vi "Window Coefficients.vi"(1 "window type":T1(ring)=enum."Hanning", 2 "window length":i32=1024) -> (0 "coefficients":dbl[](array[numeric]) format="%.2f")   [LabVIEW 2017]
uses:
  <vilib>/Analysis/4window.llb/Blackman Window (DBL).vi
  <vilib>/Analysis/4window.llb/Hamming Window (DBL).vi
  <vilib>/Analysis/4window.llb/Hanning Window (DBL).vi
  <vilib>/Analysis/baseanly.llb/Unit Vector (DBL).vi
  <vilib>/Analysis/4window.llb/AllCosWindow (DBL).vi
  <vilib>/Analysis/NI_AALBase.lvlib
  <vilib>/Analysis/NI_AALPro.lvlib
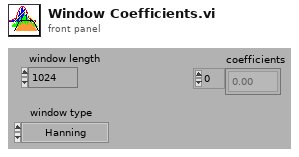
[diagram p1: front panel]
types:
  T1 = enum16{"Rectangular", "Blackman", "Hamming", "Hanning", "Gaussian"}
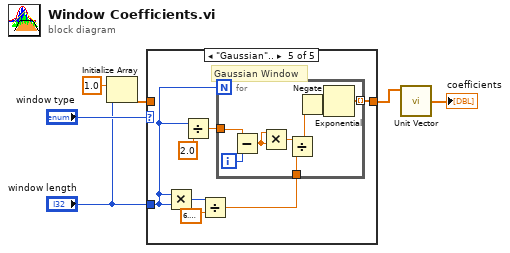
[diagram p0: block diagram]
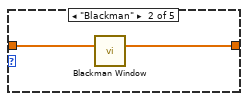
[diagram p3: hidden frame]
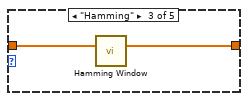
[diagram p4: hidden frame]
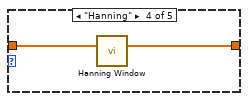
[diagram p5: hidden frame]
diagram:
  n1 = Initialize Array(1.0, "window length") -> (w4:dbl[])
  n2 = case shown="\"Gaussian\".." "window type" {
    tunnel: "window length" -> [_ _ _ _ w15]
    tunnel: [w7 w8 w10 w12 w17] -> w2
    tunnel: w4 -> [w7 w9 w11 w13 _]
    frame "Rectangular" {
      # "Rectangular"
    }
    frame "Blackman" {
      n3 = call-poly <vilib>:"Blackman Window.vi"("X"=w9) -> ("Windowed X"=w8:dbl[])  [unwired: 1 out]
    }
    frame "Hamming" {
      n4 = call-poly <vilib>:"Hamming Window.vi"("X"=w11) -> ("Windowed X"=w10:dbl[])  [unwired: 1 out]
    }
    frame "Hanning" {
      n5 = call-poly <vilib>:"Hanning Window.vi"("X"=w13) -> ("Windowed X"=w12:dbl[])  [unwired: 1 out]
    }
    frame "Gaussian".. {
      # "Gaussian Window"
      n6 = Multiply(x=w15, y=w15) -> (x*y=w16:i32)
      n7 = Divide(x=w15, y=2.0) -> (x/y=w19:dbl)
      n8 = Divide(x=w16, y=6.283185307179586) -> (x/y=w18:dbl)
      n9 = for {
        N: w15 -> [_]
        tunnel: [w23] -> w17 mode=indexing
        tunnel: w18 -> [w26]
        tunnel: w19 -> [w21]
        i -> [w28]
        n10 = Subtract(x=w21, y=w28) -> (x-y=w22:dbl)
        n11 = Multiply(x=w22, y=w22) -> (x*y=w27:dbl)
        n12 = Divide(x=w27, y=w26) -> (x/y=w25:dbl)
        n13 = Negate(x=w25) -> (-x=w24:dbl)
        n14 = Exponential(1:w24) -> (0:w23:dbl)
      }
    }
  }
  n15 = call-poly <vilib>:"Unit Vector.vi"("Input Vector"=w2) -> ("Unit Vector"=→"coefficients":dbl[])  [unwired: 8 in, 2 out]
